vi "ParaAdd.vi"(11 "段名":string) -> ()   [LabVIEW 2020]
uses:
  <vilib>/Utility/config.llb/Write Key (Boolean).vi
  <vilib>/Utility/config.llb/NI_LVConfig.lvlib
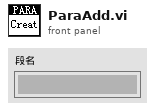
[diagram p1: front panel]
types:
  T1 = typedef "NI_LVConfig.lvlib/Config Data RefNum.ctl" = refnum<k1>
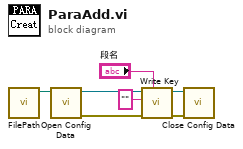
[diagram p0: block diagram]
diagram:
  n1 = call "FilePath.vi"() -> ("添加的路径"=w4:path)  [unwired: 11 in]
  n2 = call <vilib>:"Open Config Data.vi"("configuration file path"=w4) -> ("error out"=w5:errorcluster, "refnum"=w7:T1)  [unwired: 8 in, 1 out]
  n3 = call-poly <vilib>:"Write Key.vi"("section"="段名", "error in (no error)"=w5, "key"="", "refnum"=w7) -> ("error out"=w2:errorcluster, "refnum out"=w3:T1)  [unwired: 5 in, 1 out]
  n4 = call <vilib>:"Close Config Data.vi"("error in (no error)"=w2, "refnum"=w3) -> ()  [unwired: 8 in, 2 out]
